vi "create default alias.vi"(8 "error in":errorcluster, 11 "CEF_Configuration in":refnum<class "CEF_serializable configuration.lvclass">) -> (0 "error out":errorcluster, 2 "default alias":string, 3 "CEF_Configuration out":refnum<class "CEF_serializable configuration.lvclass">)   [LabVIEW 2025, in "CEF.lvlib" / "CEF_serializable configuration.lvclass"]
doc: "Copyright 2017 National Instruments Corporation\n\nLicensed under the Apache License, Version 2.0 (the \"License\"); you may not use this file except in compliance with the License. You may obtain a copy of the License at http://www.apache.org/licenses/LICENSE-2.0\nUnless required by applicable law or agreed to in writing, software distributed under the License is distributed on an \"AS IS\" BASIS, WITHOUT WARRANTIES OR CONDITIONS OF ANY KIND, either express or implied. See the License for the specific language governing permissions and limitations under the License."
uses:
  CEF_serializable configuration.lvclass
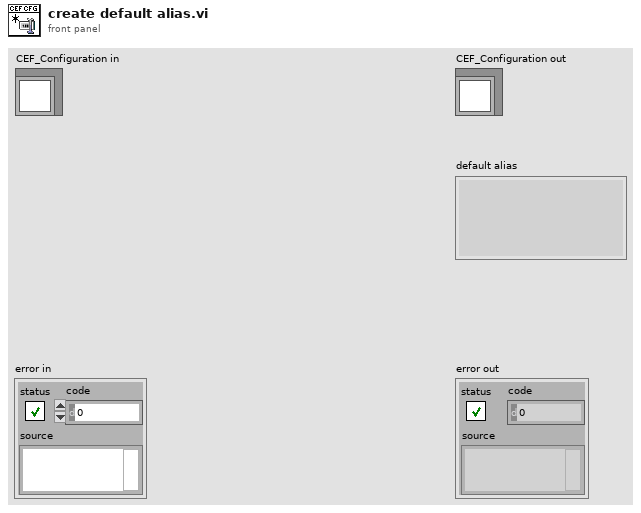
[diagram p1: front panel]
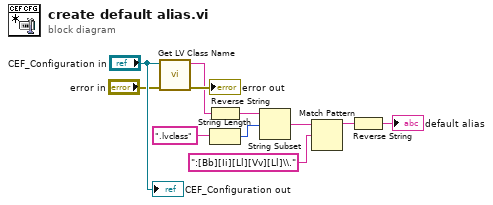
[diagram p0: block diagram]
diagram:
  n1 = call <vilib>:"Get LV Class Name.vi"("error in (no error)"="error in", "object"="CEF_Configuration in") -> ("error out"=→"error out":errorcluster, "class name"=w8:string)  [unwired: 8 in]
  n2 = Reverse String(1:w8) -> (0:w7:string)
  n3 = String Length(string=".lvclass") -> (length=w5:i32)
  n4 = String Subset(string=w7, offset (0)=w5) -> (substring=w4:string)  [unwired: 1 in]
  n5 = Match Pattern(string=w4, regular expression=":[Bb][Ii][Ll][Vv][Ll]\\.") -> (before substring=w2:string)  [unwired: 1 in, 3 out]
  n6 = Reverse String(1:w2) -> (0:→"default alias":string)
  "CEF_Configuration out" <- "CEF_Configuration in"
